vi "SCCSup Dialog_GenMCLB_Sort.vi"(6 "treat as number?":bool, 8 "error in (no error)":errorcluster, 9 "Clicked Col Hdr":i32, 11 "MCListbox Refnum":refnum<vi>) -> (0 "error out":errorcluster)   [LabVIEW 2020]
doc: "This VI sorts a multicolumn listbox when you click a column header. Click a column hearder once to sort that column in ascending order. Click the header again to sort the column in descending order. The VI reorders all other columns to maintain row integrity. You can wire a multicolumn listbox control reference to this VI."
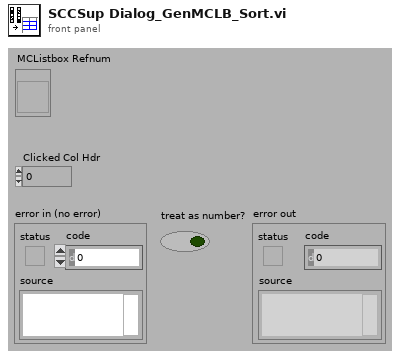
[diagram p1: front panel]
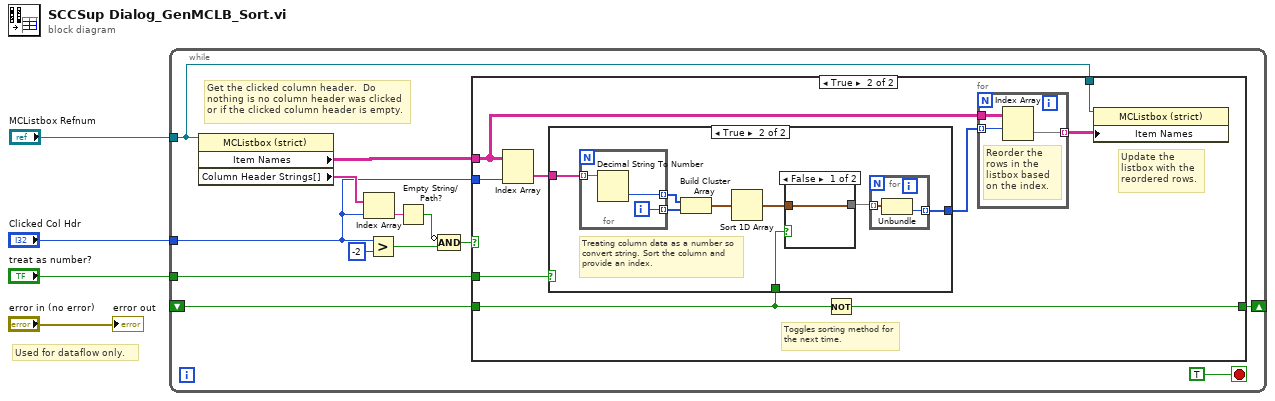
[diagram p0: block diagram]
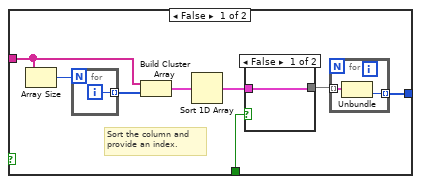
[diagram p3: hidden frame]
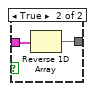
[diagram p4: hidden frame]
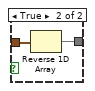
[diagram p5: hidden frame]
diagram:
  # "Used for dataflow only."
  n1 = while {
    shift-right: [w15] -> _
    shift-left: _ -> [w16]
    tunnel: "MCListbox Refnum" -> [w12]
    tunnel: "Clicked Col Hdr" -> [w7]
    tunnel: "treat as number?" -> [w5]
    stop <- TRUE stop-if-true
    # "Get the clicked column header.  Do nothing is no column header was clicked or if the clicked column header is empty."
    n2 = property class="MCListbox (strict)"(reference=w12) -> ("Item Names"=w13:string[][], "Column Header Strings[]"=w11:string[])  [unwired: 1 in, 2 out]
    n3 = Index Array(array=w11, index=w7) -> (element=w10:string)
    n4 = Greater?(x=w7, y=-2) -> (0:w9:bool)
    n5 = Empty String/Path?(string/path=w10) -> (empty?=w8:bool)
    n6 = Compound Arithmetic op=AND(invert w8, w9) -> (w6:bool)
    n7 = case shown="True" w6 {
      tunnel: w13 -> [_ w26]
      tunnel: w7 -> [_ w27]
      tunnel: w16 -> [w18 w22]
      tunnel: [w18 w25] -> w15
      tunnel: w12 -> [_ w23]
      tunnel: w5 -> [_ w19]
      frame False {
      }
      frame True {
        # "Toggles sorting method for the next time."
        # "Update the listbox with the reordered rows."
        n8 = Index Array(array=w26, index (col)=w27) -> (element=w20:string[])  [unwired: 1 in]
        n9 = case shown="True" w19 {
          tunnel: w22 -> [w32 w46]
          tunnel: [w31 w45] -> w21
          tunnel: w20 -> [w28 w44]
          frame False {
            # "Sort the column and provide an index."
            n10 = Array Size(array=w28) -> (size(s)=w29:i32)
            n11 = for {
              N: w29 -> [_]
              tunnel: [w36] -> w30 mode=indexing
              i -> [w36]
            }
            n12 = Build Cluster Array ("Index & Bundle Cluster Array")(w28, w30) -> (w33:cluster{string, i32}[])
            n13 = Sort 1D Array(array=w33) -> (sorted array=w34:cluster{string, i32}[])
            n14 = case shown="False" w32 {
              tunnel: w34 -> [w37 w39]
              tunnel: [w37 w38] -> w35
              frame False {
              }
              frame True {
                n15 = Reverse 1D Array(array=w39) -> (reversed array=w38:cluster{string, i32}[])
              }
            }
            n16 = for {
              tunnel: w35 -> [w41] mode=indexing
              tunnel: [w40] -> w31 mode=indexing
              n17 = Unbundle(w41) -> (w40:i32)  [unwired: 1 out]
            }
          }
          frame True {
            # "Treating column data as a number so convert string. Sort the column and provide an index."
            n18 = for {
              tunnel: w44 -> [w52] mode=indexing
              tunnel: [w51] -> w43 mode=indexing
              tunnel: [w50] -> w42 mode=indexing
              i -> [w50]
              n19 = Decimal String To Number(string=w52) -> (number=w51:i32)  [unwired: 2 in, 1 out]
            }
            n20 = Build Cluster Array ("Index & Bundle Cluster Array")(w43, w42) -> (w47:cluster{i32, i32}[])
            n21 = Sort 1D Array(array=w47) -> (sorted array=w48:cluster{i32, i32}[])
            n22 = case shown="False" w46 {
              tunnel: w48 -> [w53 w55]
              tunnel: [w53 w54] -> w49
              frame False {
              }
              frame True {
                n23 = Reverse 1D Array(array=w55) -> (reversed array=w54:cluster{i32, i32}[])
              }
            }
            n24 = for {
              tunnel: w49 -> [w57] mode=indexing
              tunnel: [w56] -> w45 mode=indexing
              n25 = Unbundle(w57) -> (w56:i32)  [unwired: 1 out]
            }
          }
        }
        n26 = Not(x=w22) -> (.not. x?=w25:bool)
        n27 = for {
          tunnel: w21 -> [w59] mode=indexing
          tunnel: w26 -> [w60]
          tunnel: [w58] -> w24 mode=indexing
          # "Reorder the rows in the listbox based\non the index."
          n28 = Index Array(array=w60, index (row)=w59) -> (element=w58:string[])  [unwired: 1 in]
        }
        n29 = property class="MCListbox (strict)"(reference=w23, "Item Names"=w24) -> ()  [unwired: 1 in, 2 out]
      }
    }
  }
  "error out" <- "error in (no error)"
